vi "Translate.vi"(10 "Message In":refnum<class "MSG.lvclass">, 11 "Translator in":refnum<class "SubstututeMessage.lvclass">) -> (2 "Translated Message":refnum<class "MSG.lvclass">, 3 "Translator out":refnum<class "SubstututeMessage.lvclass">)   [LabVIEW 2011, in "Messenging.lvlib" / "SubstututeMessage.lvclass"]
uses:
  SubstututeMessage.lvclass
  TextVarientMessage/MSG.lvclass
  SubstututeMessage.lvclass/SubstututeMessage.ctl
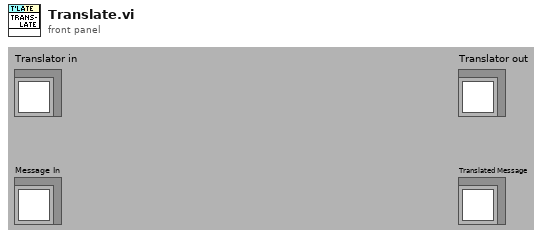
[diagram p1: front panel]
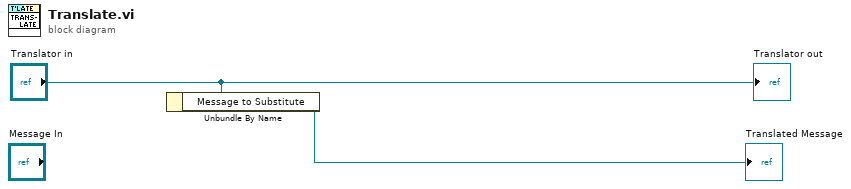
[diagram p0: block diagram]
diagram:
  n1 = Unbundle By Name("Translator in") -> ("Message to Substitute"=→"Translated Message":refnum<class "MSG.lvclass">)
  "Translator out" <- "Translator in"
